vi "rad_Convert Item Strings to FPGA Properties.vi"(11 "ItemNames":string[](array[string])) -> (3 "FPGA Properties":T1)   [LabVIEW 2013]
uses:
  TypeDefs/rad_FPGA Flash Properties.ctl
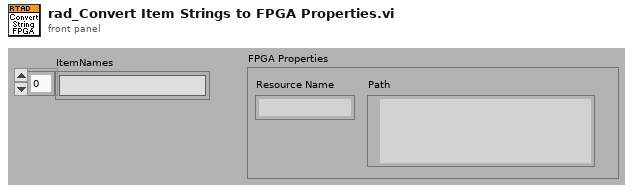
[diagram p1: front panel]
types:
  T1 = typedef "rad_FPGA Flash Properties.ctl" = cluster{"Resource Name":string, "Path":path}
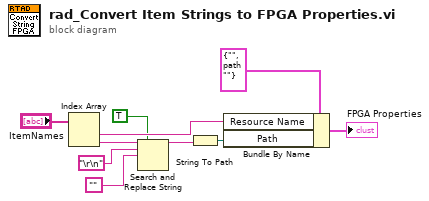
[diagram p0: block diagram]
diagram:
  n1 = Index Array(array="ItemNames") -> (element #1=w10:string, element #2=w5:string)  [unwired: 2 in]
  n2 = Search and Replace String(replace all?=TRUE ("replace all? (F)"), input string=w5, search string="\r\n", replace string="") -> (result string=w1:string)  [unwired: 4 in, 3 out]
  n3 = String To Path(string=w1) -> (path=w9:path)
  n4 = Bundle By Name(cluster=T1 {"Resource Name"="", "Path"=path ""} ("FPGA Properties"), "Resource Name"=w10, "Path"=w9) -> (→"FPGA Properties":T1)
